vi "Summarize Motion2.vi"(6 "time log":refnum<file>, 8 "external stop":refnum<vi>, 9 "motion log":refnum<file>, 10 "centroid log":refnum<file>, 11 "roi data cluster":T1={[0, 0, 1280, 960], [{"Contour Type"=0, "ROI Type"=12, [70, 141, 164, 235, 270302]}, {"Contour Type"=0, "ROI Type"=12, [70, 236, 164, 330, 270302]}, {"Contour Type"=0, "ROI Type"=12, [71, 331, 165, 425, 270302]}, {"Contour Type"=0, "ROI Type"=12, [72, 426, 166, 520, 270302]}, {"Contour Type"=0, "ROI Type"=12, [72, 520, 166, 614, 270302]}, {"Contour Type"=0, "ROI Type"=12, [72, 615, 166, 709, 270302]}, {"Contour Type"=0, "ROI Type"=12, [73, 710, 167, 804, 270302]}, {"Contour Type"=0, "ROI Type"=12, [74, 805, 168, 899, 270302]}, {"Contour Type"=0, "ROI Type"=12, [165, 140, 259, 234, 270302]}, {"Contour Type"=0, "ROI Type"=12, [165, 235, 259, 329, 270302]}, {"Contour Type"=0, "ROI Type"=12, [166, 330, 260, 424, 270302]}, {"Contour Type"=0, "ROI Type"=12, [166, 425, 260, 519, 270302]}, {"Contour Type"=0, "ROI Type"=12, [167, 520, 261, 614, 270302]}, {"Contour Type"=0, "ROI Type"=12, [167, 615, 261, 709, 270302]}, {"Contour Type"=0, "ROI Type"=12, [168, 710, 262, 804, 270302]}, {"Contour Type"=0, "ROI Type"=12, [168, 805, 262, 899, 270302]}, {"Contour Type"=0, "ROI Type"=12, [260, 140, 354, 234, 270302]}, {"Contour Type"=0, "ROI Type"=12, [260, 235, 354, 329, 270302]}, {"Contour Type"=0, "ROI Type"=12, [260, 330, 354, 424, 270302]}, {"Contour Type"=0, "ROI Type"=12, [261, 425, 355, 519, 270302]}, {"Contour Type"=0, "ROI Type"=12, [262, 520, 356, 614, 270302]}, {"Contour Type"=0, "ROI Type"=12, [262, 614, 356, 708, 270302]}, {"Contour Type"=0, "ROI Type"=12, [262, 709, 356, 803, 270302]}, {"Contour Type"=0, "ROI Type"=12, [263, 804, 357, 898, 270302]}, {"Contour Type"=0, "ROI Type"=12, [354, 140, 448, 234, 270302]}, {"Contour Type"=0, "ROI Type"=12, [355, 234, 449, 328, 270302]}, {"Contour Type"=0, "ROI Type"=12, [355, 329, 449, 423, 270302]}, {"Contour Type"=0, "ROI Type"=12, [356, 424, 450, 518, 270302]}, {"Contour Type"=0, "ROI Type"=12, [356, 519, 450, 613, 270302]}, {"Contour Type"=0, "ROI Type"=12, [357, 614, 451, 708, 270302]}, {"Contour Type"=0, "ROI Type"=12, [357, 709, 451, 803, 270302]}, {"Contour Type"=0, "ROI Type"=12, [358, 804, 452, 898, 270302]}, {"Contour Type"=0, "ROI Type"=12, [449, 139, 543, 233, 270302]}, {"Contour Type"=0, "ROI Type"=12, [450, 234, 544, 328, 270302]}, {"Contour Type"=0, "ROI Type"=12, [450, 329, 544, 423, 270302]}, {"Contour Type"=0, "ROI Type"=12, [450, 424, 544, 518, 270302]}, {"Contour Type"=0, "ROI Type"=12, [451, 518, 545, 612, 270302]}, {"Contour Type"=0, "ROI Type"=12, [452, 613, 546, 707, 270302]}, {"Contour Type"=0, "ROI Type"=12, [452, 708, 546, 802, 270302]}, {"Contour Type"=0, "ROI Type"=12, [452, 803, 546, 897, 270302]}, {"Contour Type"=0, "ROI Type"=12, [544, 138, 638, 232, 270302]}, {"Contour Type"=0, "ROI Type"=12, [544, 233, 638, 327, 270302]}, {"Contour Type"=0, "ROI Type"=12, [545, 328, 639, 422, 270302]}, {"Contour Type"=0, "ROI Type"=12, [545, 423, 639, 517, 270302]}, {"Contour Type"=0, "ROI Type"=12, [546, 518, 640, 612, 270302]}, {"Contour Type"=0, "ROI Type"=12, [546, 613, 640, 707, 270302]}, {"Contour Type"=0, "ROI Type"=12, [547, 708, 641, 802, 270302]}, {"Contour Type"=0, "ROI Type"=12, [547, 803, 641, 897, 270302]}, {"Contour Type"=0, "ROI Type"=12, [638, 138, 732, 232, 270302]}, {"Contour Type"=0, "ROI Type"=12, [639, 233, 733, 327, 270302]}, {"Contour Type"=0, "ROI Type"=12, [640, 328, 734, 422, 270302]}, {"Contour Type"=0, "ROI Type"=12, [640, 423, 734, 517, 270302]}, {"Contour Type"=0, "ROI Type"=12, [640, 518, 734, 612, 270302]}, {"Contour Type"=0, "ROI Type"=12, [641, 612, 735, 706, 270302]}, {"Contour Type"=0, "ROI Type"=12, [642, 707, 736, 801, 270302]}, {"Contour Type"=0, "ROI Type"=12, [642, 802, 736, 896, 270302]}, {"Contour Type"=0, "ROI Type"=12, [733, 138, 827, 232, 270302]}, {"Contour Type"=0, "ROI Type"=12, [734, 232, 828, 326, 270302]}, {"Contour Type"=0, "ROI Type"=12, [734, 327, 828, 421, 270302]}, {"Contour Type"=0, "ROI Type"=12, [735, 422, 829, 516, 270302]}, {"Contour Type"=0, "ROI Type"=12, [735, 517, 829, 611, 270302]}, {"Contour Type"=0, "ROI Type"=12, [736, 612, 830, 706, 270302]}, {"Contour Type"=0, "ROI Type"=12, [736, 707, 830, 801, 270302]}, {"Contour Type"=0, "ROI Type"=12, [737, 802, 831, 896, 270302]}, {"Contour Type"=0, "ROI Type"=12, [828, 137, 922, 231, 270302]}, {"Contour Type"=0, "ROI Type"=12, [828, 232, 922, 326, 270302]}, {"Contour Type"=0, "ROI Type"=12, [829, 327, 923, 421, 270302]}, {"Contour Type"=0, "ROI Type"=12, [830, 422, 924, 516, 270302]}, {"Contour Type"=0, "ROI Type"=12, [830, 516, 924, 610, 270302]}, {"Contour Type"=0, "ROI Type"=12, [830, 611, 924, 705, 270302]}, {"Contour Type"=0, "ROI Type"=12, [831, 706, 925, 800, 270302]}, {"Contour Type"=0, "ROI Type"=12, [832, 801, 926, 895, 270302]}, {"Contour Type"=0, "ROI Type"=12, [923, 136, 1017, 230, 270302]}, {"Contour Type"=0, "ROI Type"=12, [923, 231, 1017, 325, 270302]}, {"Contour Type"=0, "ROI Type"=12, [924, 326, 1018, 420, 270302]}, {"Contour Type"=0, "ROI Type"=12, [924, 421, 1018, 515, 270302]}, {"Contour Type"=0, "ROI Type"=12, [925, 516, 1019, 610, 270302]}, {"Contour Type"=0, "ROI Type"=12, [925, 611, 1019, 705, 270302]}, {"Contour Type"=0, "ROI Type"=12, [926, 706, 1020, 800, 270302]}, {"Contour Type"=0, "ROI Type"=12, [926, 801, 1020, 895, 270302]}, {"Contour Type"=0, "ROI Type"=12, [1018, 136, 1112, 230, 270302]}, {"Contour Type"=0, "ROI Type"=12, [1018, 231, 1112, 325, 270302]}, {"Contour Type"=0, "ROI Type"=12, [1018, 326, 1112, 420, 270302]}, {"Contour Type"=0, "ROI Type"=12, [1019, 421, 1113, 515, 270302]}, {"Contour Type"=0, "ROI Type"=12, [1020, 516, 1114, 610, 270302]}, {"Contour Type"=0, "ROI Type"=12, [1020, 610, 1114, 704, 270302]}, {"Contour Type"=0, "ROI Type"=12, [1020, 705, 1114, 799, 270302]}, {"Contour Type"=0, "ROI Type"=12, [1021, 800, 1115, 894, 270302]}, {"Contour Type"=0, "ROI Type"=12, [1112, 136, 1206, 230, 270302]}, {"Contour Type"=0, "ROI Type"=12, [1113, 230, 1207, 324, 270302]}, {"Contour Type"=0, "ROI Type"=12, [1113, 325, 1207, 419, 270302]}, {"Contour Type"=0, "ROI Type"=12, [1114, 420, 1208, 514, 270302]}, {"Contour Type"=0, "ROI Type"=12, [1114, 515, 1208, 609, 270302]}, {"Contour Type"=0, "ROI Type"=12, [1115, 610, 1209, 704, 270302]}, {"Contour Type"=0, "ROI Type"=12, [1115, 705, 1209, 799, 270302]}, {"Contour Type"=0, "ROI Type"=12, [1116, 800, 1210, 894, 270302]}]}) -> ()   [LabVIEW 2013]
panel:
  out "Waveform Graph":u16[][](graph)
  in  "stop":bool=TRUE
  out "centroids2":refnum<queue>
  out "motionpix2":refnum<queue>
  out "totalmotion2":refnum<queue>
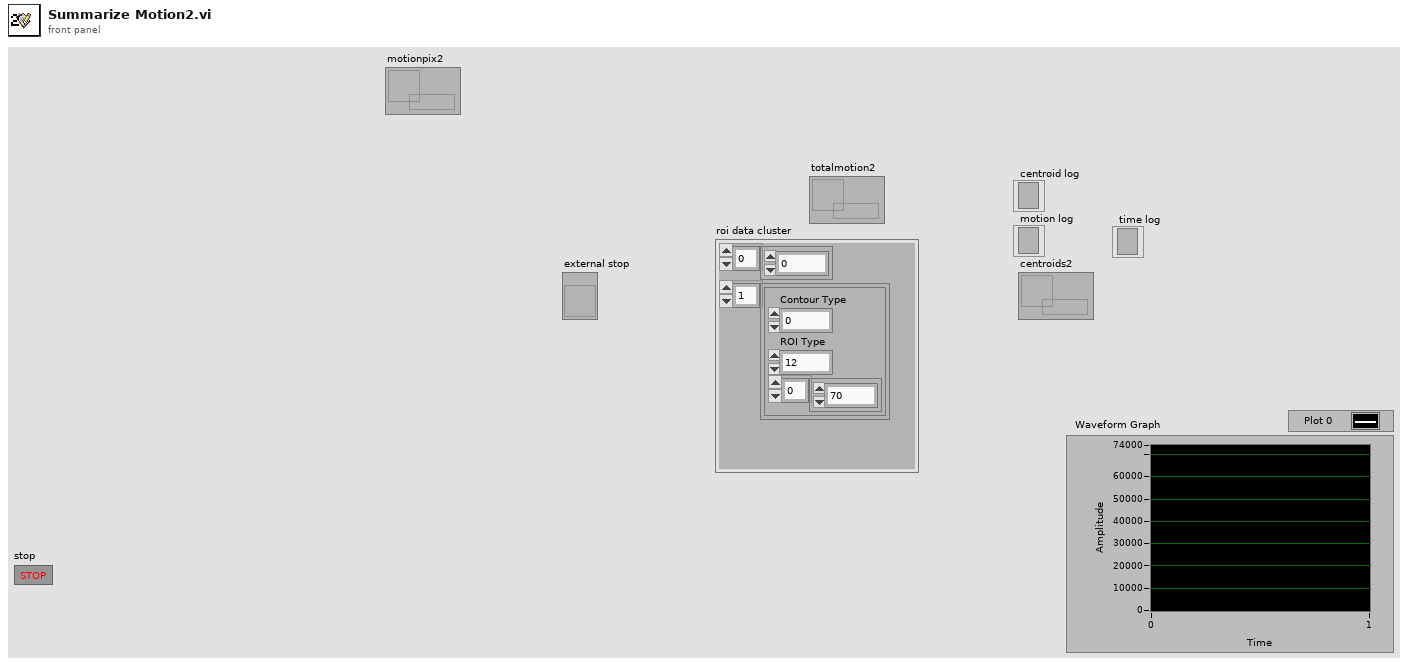
[diagram p1: front panel]
types:
  T1 = cluster{i32[], cluster{"Contour Type":u32, "ROI Type":u32, i32[]}[]}
  T2 = cluster{"Contour Type":u32, "ROI Type":u32, i32[]}[]
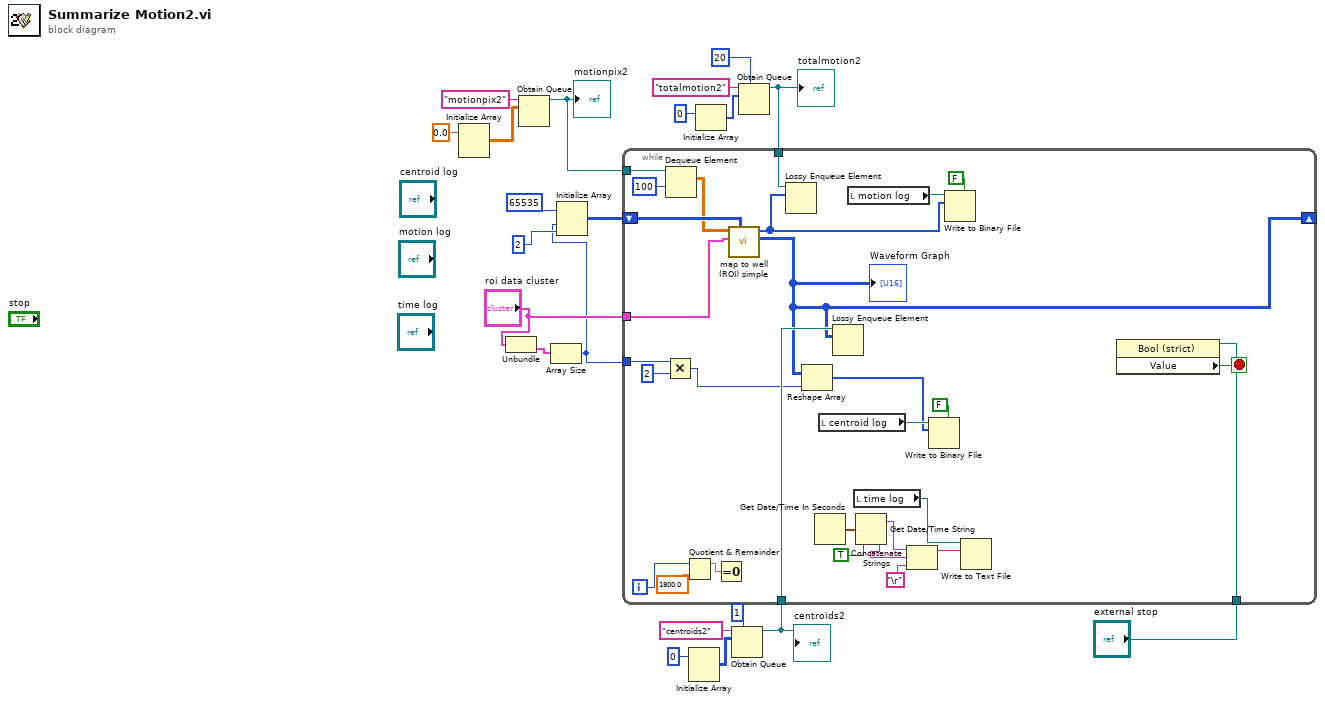
[diagram p0: block diagram]
diagram:
  n1 = Initialize Array(0.0 ("element")) -> (w11:dbl[][])  [unwired: 2 in]
  n2 = Unbundle("roi data cluster") -> (w4:T2)  [unwired: 1 out]
  n3 = Obtain Queue(name (unnamed)="motionpix2", element data type=w11) -> (queue out=w10:refnum<queue>)  [unwired: 3 in, 2 out]
  "motionpix2" <- w10
  n4 = Array Size(array=w4) -> (size(s)=w3:i32)
  n5 = Initialize Array(u16 65535 ("element"), w3, 2 ("dimension size")) -> (w18:u16[][])
  n6 = Initialize Array(u16 0 ("element")) -> (w9:u16[][])  [unwired: 2 in]
  n7 = Initialize Array(u16 0 ("element")) -> (w15:u16[])  [unwired: 1 in]
  n8 = Obtain Queue(max queue size (-1, unlimited)=1, name (unnamed)="centroids2", element data type=w9) -> (queue out=w6:refnum<queue>)  [unwired: 2 in, 2 out]
  "centroids2" <- w6
  n9 = Obtain Queue(max queue size (-1, unlimited)=20, name (unnamed)="totalmotion2", element data type=w15) -> (queue out=w14:refnum<queue>)  [unwired: 2 in, 2 out]
  "totalmotion2" <- w14
  n10 = while {
    tunnel: "external stop" -> [w50]
    shift-right: [w35] -> _
    shift-left: w18 -> [w47]
    tunnel: w14 -> [w48]
    tunnel: w10 -> [w46]
    tunnel: "roi data cluster" -> [w43]
    tunnel: w6 -> [w42]
    tunnel: w3 -> [w38]
    i -> [w39]
    stop <- w49 stop-if-true
    n11 = Multiply(x=w38, y=2) -> (x*y=w36:i32)
    n12 = Dequeue Element(queue=w46, timeout in ms (-1)=100) -> (element=w44:dbl[][])  [unwired: 1 in, 3 out]
    n13 = Quotient & Remainder(x=w39, y=1800.0) -> (x-y*floor(x/y)=w41:dbl)  [unwired: 1 out]
    n14 = Equal To 0?(x=w41) -> ()  [unwired: 1 out]
    n15 = call "map to well (ROI) simple.vi"("centroids in"=w47, "roi data cluster"=w43, "Particle Measurements (Pixels)"=w44) -> ("centroids out"=w35:u16[][], "roi total motion"=w26:u16[])  [unwired: 7 in]
    "Waveform Graph" <- w35
    n16 = Lossy Enqueue Element(queue=w48, element=w26) -> ()  [unwired: 1 in, 4 out]
    n17 = Reshape Array(w35, w36) -> (w23:u16[])
    n18 = Get Date/Time In Seconds() -> (seconds since 1Jan1904=w34:timestamp)
    n19 = local read "centroid log"() -> (w24:refnum<file>)
    n20 = Lossy Enqueue Element(queue=w42, element=w35) -> ()  [unwired: 1 in, 4 out]
    n21 = local read "motion log"() -> (w28:refnum<file>)
    n22 = local read "time log"() -> (w29:refnum<file>)
    n23 = Get Date/Time String(seconds (now)=w34, want seconds? (F)=TRUE) -> (date string=w22:string, time string=w32:string)  [unwired: 1 in]
    n24 = Concatenate Strings(w22, w32, "\r") -> (w31:string)
    n25 = Write to Binary File(file (use dialog)=w24, data=w23, 5:FALSE ("prepend array or string size? (T)")) -> ()  [unwired: 3 in, 3 out]
    n26 = Write to Binary File(file (use dialog)=w28, data=w26, 5:FALSE ("prepend array or string size? (T)")) -> ()  [unwired: 3 in, 3 out]
    n27 = Write to Text File(file (use dialog)=w29, text=w31) -> ()  [unwired: 2 in, 3 out]
    n28 = property class="Bool (strict)"(reference=w50) -> ("Value"=w49:bool)  [unwired: 1 in, 2 out]
  }
